vi "H5Tget_inpad.vi"(6 "error in (no error)":errorcluster, 9 "HDF5 Ref":T2) -> (0 "error out":errorcluster, 2 "Padding":T1 items=["H5T_PAD_ERROR"=-1, "H5T_PAD_ZERO"=0, "H5T_PAD_ONE"=1, "H5T_PAD_BACKGROUND"=2], 3 "HDF5 Ref out":T2)   [LabVIEW 2017]
doc: "Retrieves the internal padding type for unused bits in floating-point datatypes."
uses:
  <vilib>/UPVI/lvhdf5/library.llb/HDF5 Ref.ctl
  <vilib>/UPVI/lvhdf5/datatype.llb/H5T_pad_t.ctl
  <vilib>/UPVI/lvhdf5/hdf5.dll
panel:
  # "LVHDF5 Toolkit\nCopyright (c) 2005-2013 by Jason D. Sommerville\nCopyright (c) 2014 by UPVI, LLC.\n\nThis use and distribution of this file is governed by the terms found in \nLICENSE.txt distributed with this toolkit and installed at\n <user.lib>\\_lvhdf5\\LICENSE.txt"
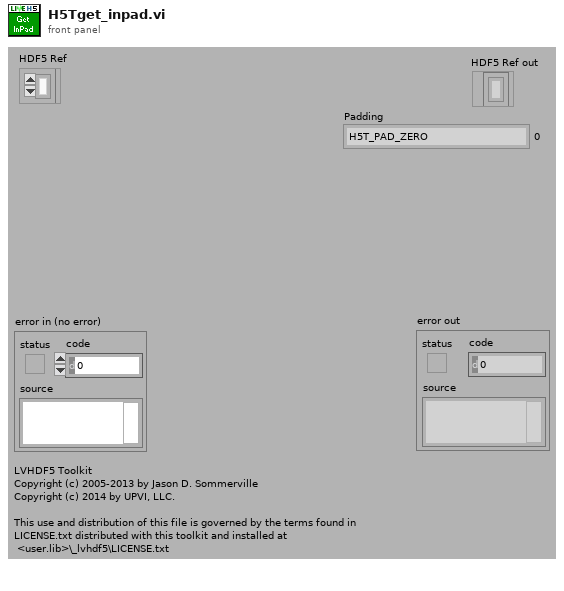
[diagram p1: front panel]
types:
  T1 = typedef "H5T_pad_t.ctl" = i32
  T2 = typedef "HDF5 Ref.ctl" = refnum<k1>
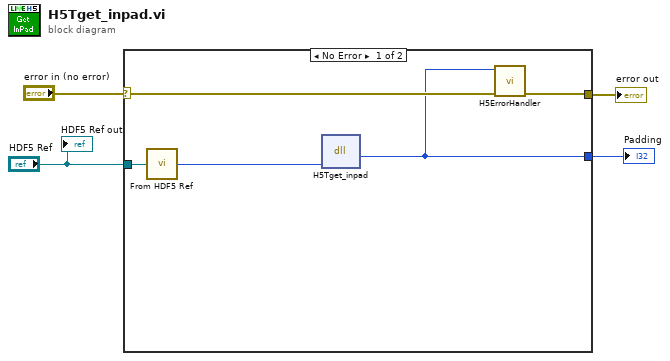
[diagram p0: block diagram]
diagram:
  n1 = case shown="No Error" "error in (no error)" {
    selector: "error in (no error)" -> [w9 w10]
    tunnel: [w8 w10] -> w3
    tunnel: "HDF5 Ref" -> [w7 _]
    tunnel: [w5 _] -> w1
    frame No Error {
      n2 = call <vilib>:"From HDF5 Ref.vi"("HDF5 Ref"=w7) -> ("I32"=w6:i32)
      n3 = dll-call lib="C:/Program Files/National Instruments/LabVIEW 2017/vi.lib/UPVI/lvhdf5/hdf5.dll" fn="H5Tget_inpad"("loc_id"=w6) -> (w5:i32)  [unwired: 4 in, 2 out]
      n4 = call <vilib>:"H5ErrorHandler.vi"("error in (no error)"=w9, "herr_t"=w5) -> ("error out"=w8:errorcluster)  [unwired: 3 in, 4 out]
    }
    frame Error {
    }
  }
  "error out" <- w3
  "Padding" <- w1
  "HDF5 Ref out" <- "HDF5 Ref"
